vi "Gen Main.vi"(10 "Data Type DVRs":T1, 11 "Config Folder":path) -> ()   [LabVIEW 2018]
uses:
  <vilib>/ORNL/CSEISMIC DDS/CSEISMIC DDS Base/Data Types/Controls/DeviceID.ctl
  Controls/DDS State.ctl
  Controls/Data Type DVRs.ctl
  Controls/Generation Mode Loop Selector.ctl
  <vilib>/ORNL/CSEISMIC DDS/CSEISMIC DDS Base/Data Types/DER_setGenerationMode.ctl
  <vilib>/ORNL/CSEISMIC DDS/CSEISMIC DDS Base/Data Types/Controls/Generation Mode.ctl
  Controls/GenerationMode.ctl
  <vilib>/ORNL/CSEISMIC DDS/CSEISMIC DDS Base/Data Types/IED_Status.ctl
  <vilib>/ORNL/CSEISMIC DDS/CSEISMIC DDS Base/Data Types/Controls/Timestamp.ctl
  <vilib>/ORNL/CSEISMIC DDS/CSEISMIC DDS Base/Data Types/DER_Control.ctl
  <vilib>/ORNL/CSEISMIC DDS/CSEISMIC DDS Base/Data Types/DER_SetPointP.ctl
  <vilib>/ORNL/CSEISMIC DDS/CSEISMIC DDS Base/Data Types/DER_SetPointQ.ctl
  <vilib>/ORNL/CSEISMIC DDS/CSEISMIC DDS Base/Data Types/DER_SetPointF.ctl
  <vilib>/ORNL/CSEISMIC DDS/CSEISMIC DDS Base/Data Types/DER_VF.ctl
  <vilib>/ORNL/CSEISMIC DDS/CSEISMIC DDS Base/Data Types/DER_SetPointV.ctl
  <vilib>/ORNL/CSEISMIC DDS/CSEISMIC DDS Base/Data Types/DER_Measurement.ctl
  <vilib>/ORNL/CSEISMIC DDS/CSEISMIC DDS Base/Data Types/DER_Status.ctl
  <vilib>/ORNL/CSEISMIC DDS/CSEISMIC DDS Base/Data Types/Controls/DroopCurve.ctl
  401ef75d-4035-4dac-a689-94d2924f7ced.vi
  ab331fe9-b04e-4426-a1fd-c0893e9cbbab.vi
  3f4c0bec-be85-4757-afce-5fb011e1cb8b.vi
  89cbe241-b989-4977-afe6-711c5348a61b.vi
  9317fa08-e0dc-4cca-bb56-0a6db7703743.vi
  886c343d-5278-4dca-8794-94646f0fb70e.vi
  c2bfef2e-7af0-43a2-a662-0b996137247f.vi
  dc0c45d3-0bd6-4f4b-910c-54dfdd797161.vi
  e30d74d1-6a2d-4639-bc13-a8367489f367.vi
  906873a0-33da-4e1e-a43f-91631b103c02.vi
  1debb0a8-2f31-4473-8656-42ab50186c7a.vi
  21a46faf-e81a-4fcd-8f80-ead2e695587f.vi
  38cde540-623b-4de9-a38b-94f214654436.vi
  4f1983b4-d265-4997-ba90-a7128872a41b.vi
  66ace3ea-5fe4-466d-8ac4-009297ea2c08.vi
  Global Variables/Stop (Global).vi
  Global Variables/Measurements (Global).vi
  Global Variables/DDS States (Global).vi
  <vilib>/ORNL/CSEISMIC DDS/CSEISMIC DDS Base/CSEISMIC DDS.lvclass
panel:
  out "P_ref":sgl
  out "Q_ref":sgl
  out "P_meas":sgl
  out "Vf Control":bool
  out "Q_meas":sgl
  out "f_islanded":fxp<+,20,6>
  out "Vq_ref":sgl
  out "Is VF Device?":bool
  in  "Ramp Rate (W)":sgl=5000.0
  out "MicrogridID":u8
  out "Error in DDS Loop":bool
  out "DDS Loop error out":errorcluster
  out "DDS State":T2=enum."Shutdown"
  out "DDS loop time":u32=103
  out "DDS Indicators":T3
  out "Error in Generation Mode Loop":bool
  out "error out GenMode Loop":errorcluster
  out "DDS state m/c loop time":u32=100
  out "DeviceID":T4
  out "Enable INV A":bool
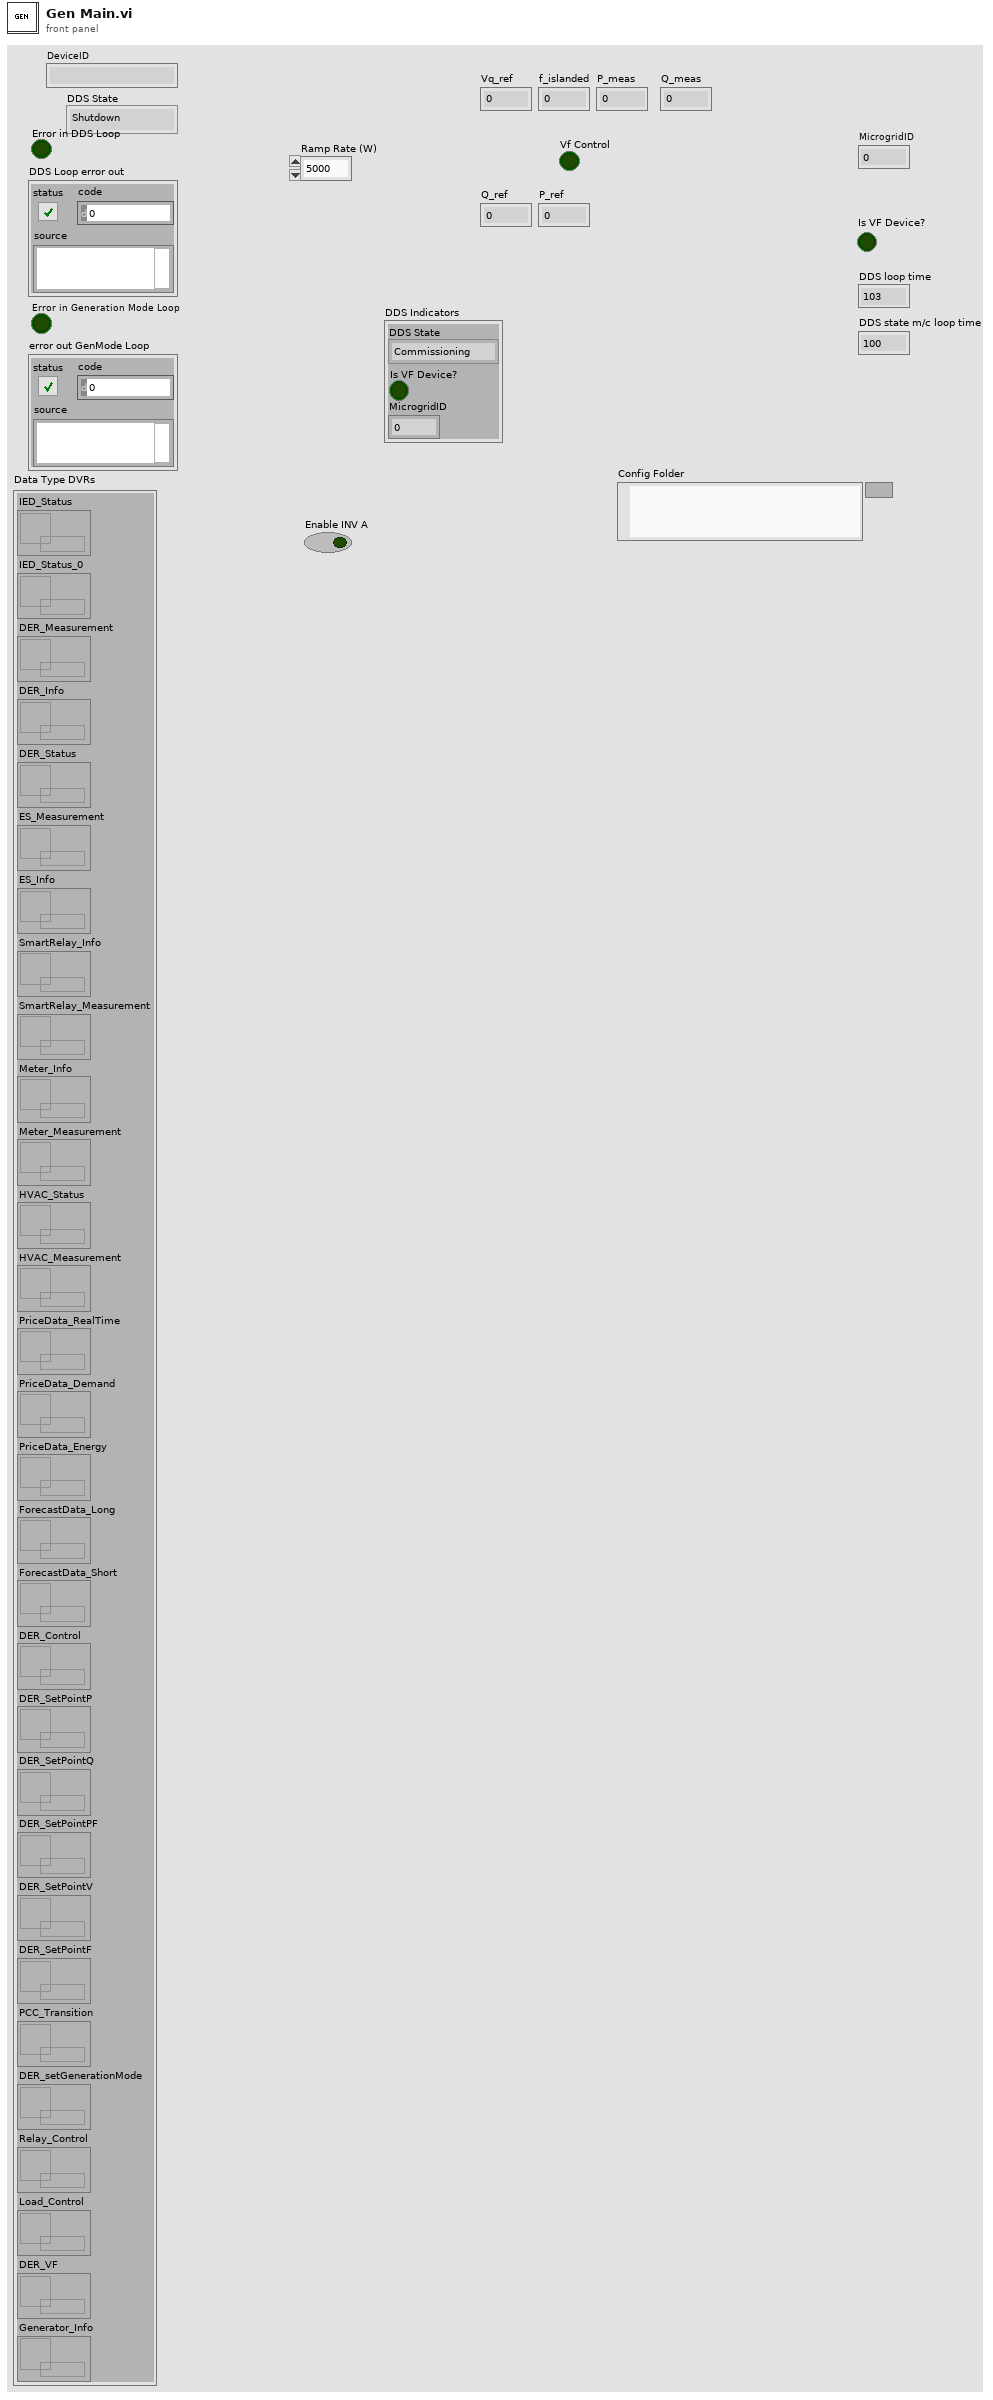
[diagram p1: front panel]
types:
  T1 = typedef "Data Type DVRs.ctl" = cluster{"IED_Status":refnum<data-value>, "IED_Status_0":refnum<data-value>, "DER_Measurement":refnum<data-value>, "DER_Info":refnum<data-value>, "DER_Status":refnum<data-value>, "ES_Measurement":refnum<data-value>, "ES_Info":refnum<data-value>, "SmartRelay_Info":refnum<data-value>, "SmartRelay_Measurement":refnum<data-value>, "Meter_Info":refnum<data-value>, "Meter_Measurement":refnum<data-value>, "HVAC_Status":refnum<data-value>, "HVAC_Measurement":refnum<data-value>, "PriceData_RealTime":refnum<data-value>, "PriceData_Demand":refnum<data-value>, "PriceData_Energy":refnum<data-value>, "ForecastData_Long":refnum<data-value>, "ForecastData_Short":refnum<data-value>, "DER_Control":refnum<data-value>, "DER_SetPointP":refnum<data-value>, "DER_SetPointQ":refnum<data-value>, "DER_SetPointPF":refnum<data-value>, "DER_SetPointV":refnum<data-value>, "DER_SetPointF":refnum<data-value>, "PCC_Transition":refnum<data-value>, "DER_setGenerationMode":refnum<data-value>, "Relay_Control":refnum<data-value>, "Load_Control":refnum<data-value>, "DER_VF":refnum<data-value>, "Generator_Info":refnum<data-value>}
  T2 = typedef "DDS State.ctl" = enum16{"Commissioning", "CheckID", "InitDDS", "ReadDDS", "WriteDDS", "CheckClose", "Close", "Shutdown"}
  T3 = cluster{"DDS State":T2, "Is VF Device?":bool, "MicrogridID":u8}
  T4 = typedef "CSEISMIC DDS.lvlib/CSEISMIC DDS.lvclass/DeviceID.ctl" = string
  T5 = typedef "Generation Mode Loop Selector.ctl" = enum16{"Commissioning", "Start", "Active", "VF Device", "Hold", "Close References", "Shutdown"}
  T6 = typedef "Scaling Coefficients Cluster.ctl" = cluster{"Measurements":T7, "Setpoints":T8}
  T7 = typedef "Scaling Coefficients Measurements.ctl" = cluster{"Current":dbl, "Voltage":dbl, "Real Power":dbl, "Reactive Power":dbl, "SOC":dbl}
  T8 = typedef "Scaling Coefficients Setpoints.ctl" = cluster{"Voltage":dbl, "Frequency":dbl, "Real Power":dbl, "Reactive Power":dbl}
  T9 = typedef "CSEISMIC DDS.lvlib/CSEISMIC DDS.lvclass/DER_Info.ctl" = cluster{"DeviceID":T4, "LineConfig":u8[], "NominalVoltage(V)":dbl, "PowerRating(kVA)":dbl, "VFControl":bool, "PControl":bool, "QControl":bool, "PFControl":bool, "PVControl":bool, "Droop":bool, "DroopConfigurable":bool, "Unbalanced":bool}
  T10 = typedef "CSEISMIC DDS.lvlib/CSEISMIC DDS.lvclass/Generator_Info.ctl" = cluster{"DeviceID":T4, "Voltage (V)":dbl, "MinimumPower (kVA)":dbl, "EnergyRating (kWh)":dbl, "RampRate (kW/s)":dbl, "MaxPowerFactorLeading":dbl, "MaxPowerFactorLagging":dbl, "EfficiencyCurve":T11, "StartCost":dbl, "FuelCost":dbl, "StartTime (s)":dbl}
  T11 = typedef "CSEISMIC DDS.lvlib/CSEISMIC DDS.lvclass/EfficiencyCurve.ctl" = cluster{"Power (kW)":dbl[], "Efficiency (%)":dbl[]}
  T12 = typedef "CSEISMIC DDS.lvlib/CSEISMIC DDS.lvclass/DER_setGenerationMode.ctl" = cluster{"DeviceID":T4, "Mode":T13}
  T13 = typedef "CSEISMIC DDS.lvlib/CSEISMIC DDS.lvclass/Generation Mode.ctl" = enum32{"Invalid", "PQ", "Droop", "PV", "PF", "VF"}
  T14 = typedef "GenerationMode.ctl" = enum32{"Invalid", "PQ", "Droop", "PV", "PF", "VF"}
  T15 = typedef "CSEISMIC DDS.lvlib/CSEISMIC DDS.lvclass/Timestamp.ctl" = cluster{"Seconds":u64, "Remainder":u64}
  T16 = typedef "CSEISMIC DDS.lvlib/CSEISMIC DDS.lvclass/IED_Status.ctl" = cluster{"DeviceID":T4, "Timestamp":T15, "MicrogridID":u8, "Active":bool, "Inactive":bool, "Error":i32, "Fault":bool, "ErrorString":string}
  T17 = typedef "CSEISMIC DDS.lvlib/CSEISMIC DDS.lvclass/DER_SetPointV.ctl" = cluster{"DeviceID":T4, "Voltage (V)":dbl}
  T18 = typedef "CSEISMIC DDS.lvlib/CSEISMIC DDS.lvclass/DER_VF.ctl" = cluster{"DeviceID":T4}
  T19 = typedef "CSEISMIC DDS.lvlib/CSEISMIC DDS.lvclass/DER_SetPointF.ctl" = cluster{"DeviceID":T4, "Frequency (Hz)":dbl}
  T20 = typedef "CSEISMIC DDS.lvlib/CSEISMIC DDS.lvclass/DER_SetPointQ.ctl" = cluster{"DeviceID":T4, "ReactivePower (kVAR)":dbl[]}
  T21 = typedef "CSEISMIC DDS.lvlib/CSEISMIC DDS.lvclass/DER_SetPointP.ctl" = cluster{"DeviceID":T4, "RealPower (kW)":dbl[]}
  T22 = typedef "CSEISMIC DDS.lvlib/CSEISMIC DDS.lvclass/DER_Control.ctl" = cluster{"DeviceID":T4, "Activate":bool, "Deactivate":bool}
  T23 = typedef "CSEISMIC DDS.lvlib/CSEISMIC DDS.lvclass/DER_Status.ctl" = cluster{"DeviceID":T4, "VFControl":bool, "PControl":bool, "QControl":bool, "PFControl":bool, "PVControl":bool, "Droop":bool, "Unbalanced":bool, "MicrogridVF":bool, "RealDroop(kW)":T24, "ReactiveDroop(kVar)":T24}
  T24 = typedef "CSEISMIC DDS.lvlib/CSEISMIC DDS.lvclass/DroopCurve.ctl" = cluster{"XMin":dbl, "XMax":dbl, "YMin":dbl, "YMax":dbl}
  T25 = typedef "CSEISMIC DDS.lvlib/CSEISMIC DDS.lvclass/DER_Measurement.ctl" = cluster{"DeviceID":T4, "Voltage":dbl[], "Current":dbl[], "RealPower":dbl[], "ReactivePower":dbl[], "LineConfig":u8[], "Frequency":dbl}
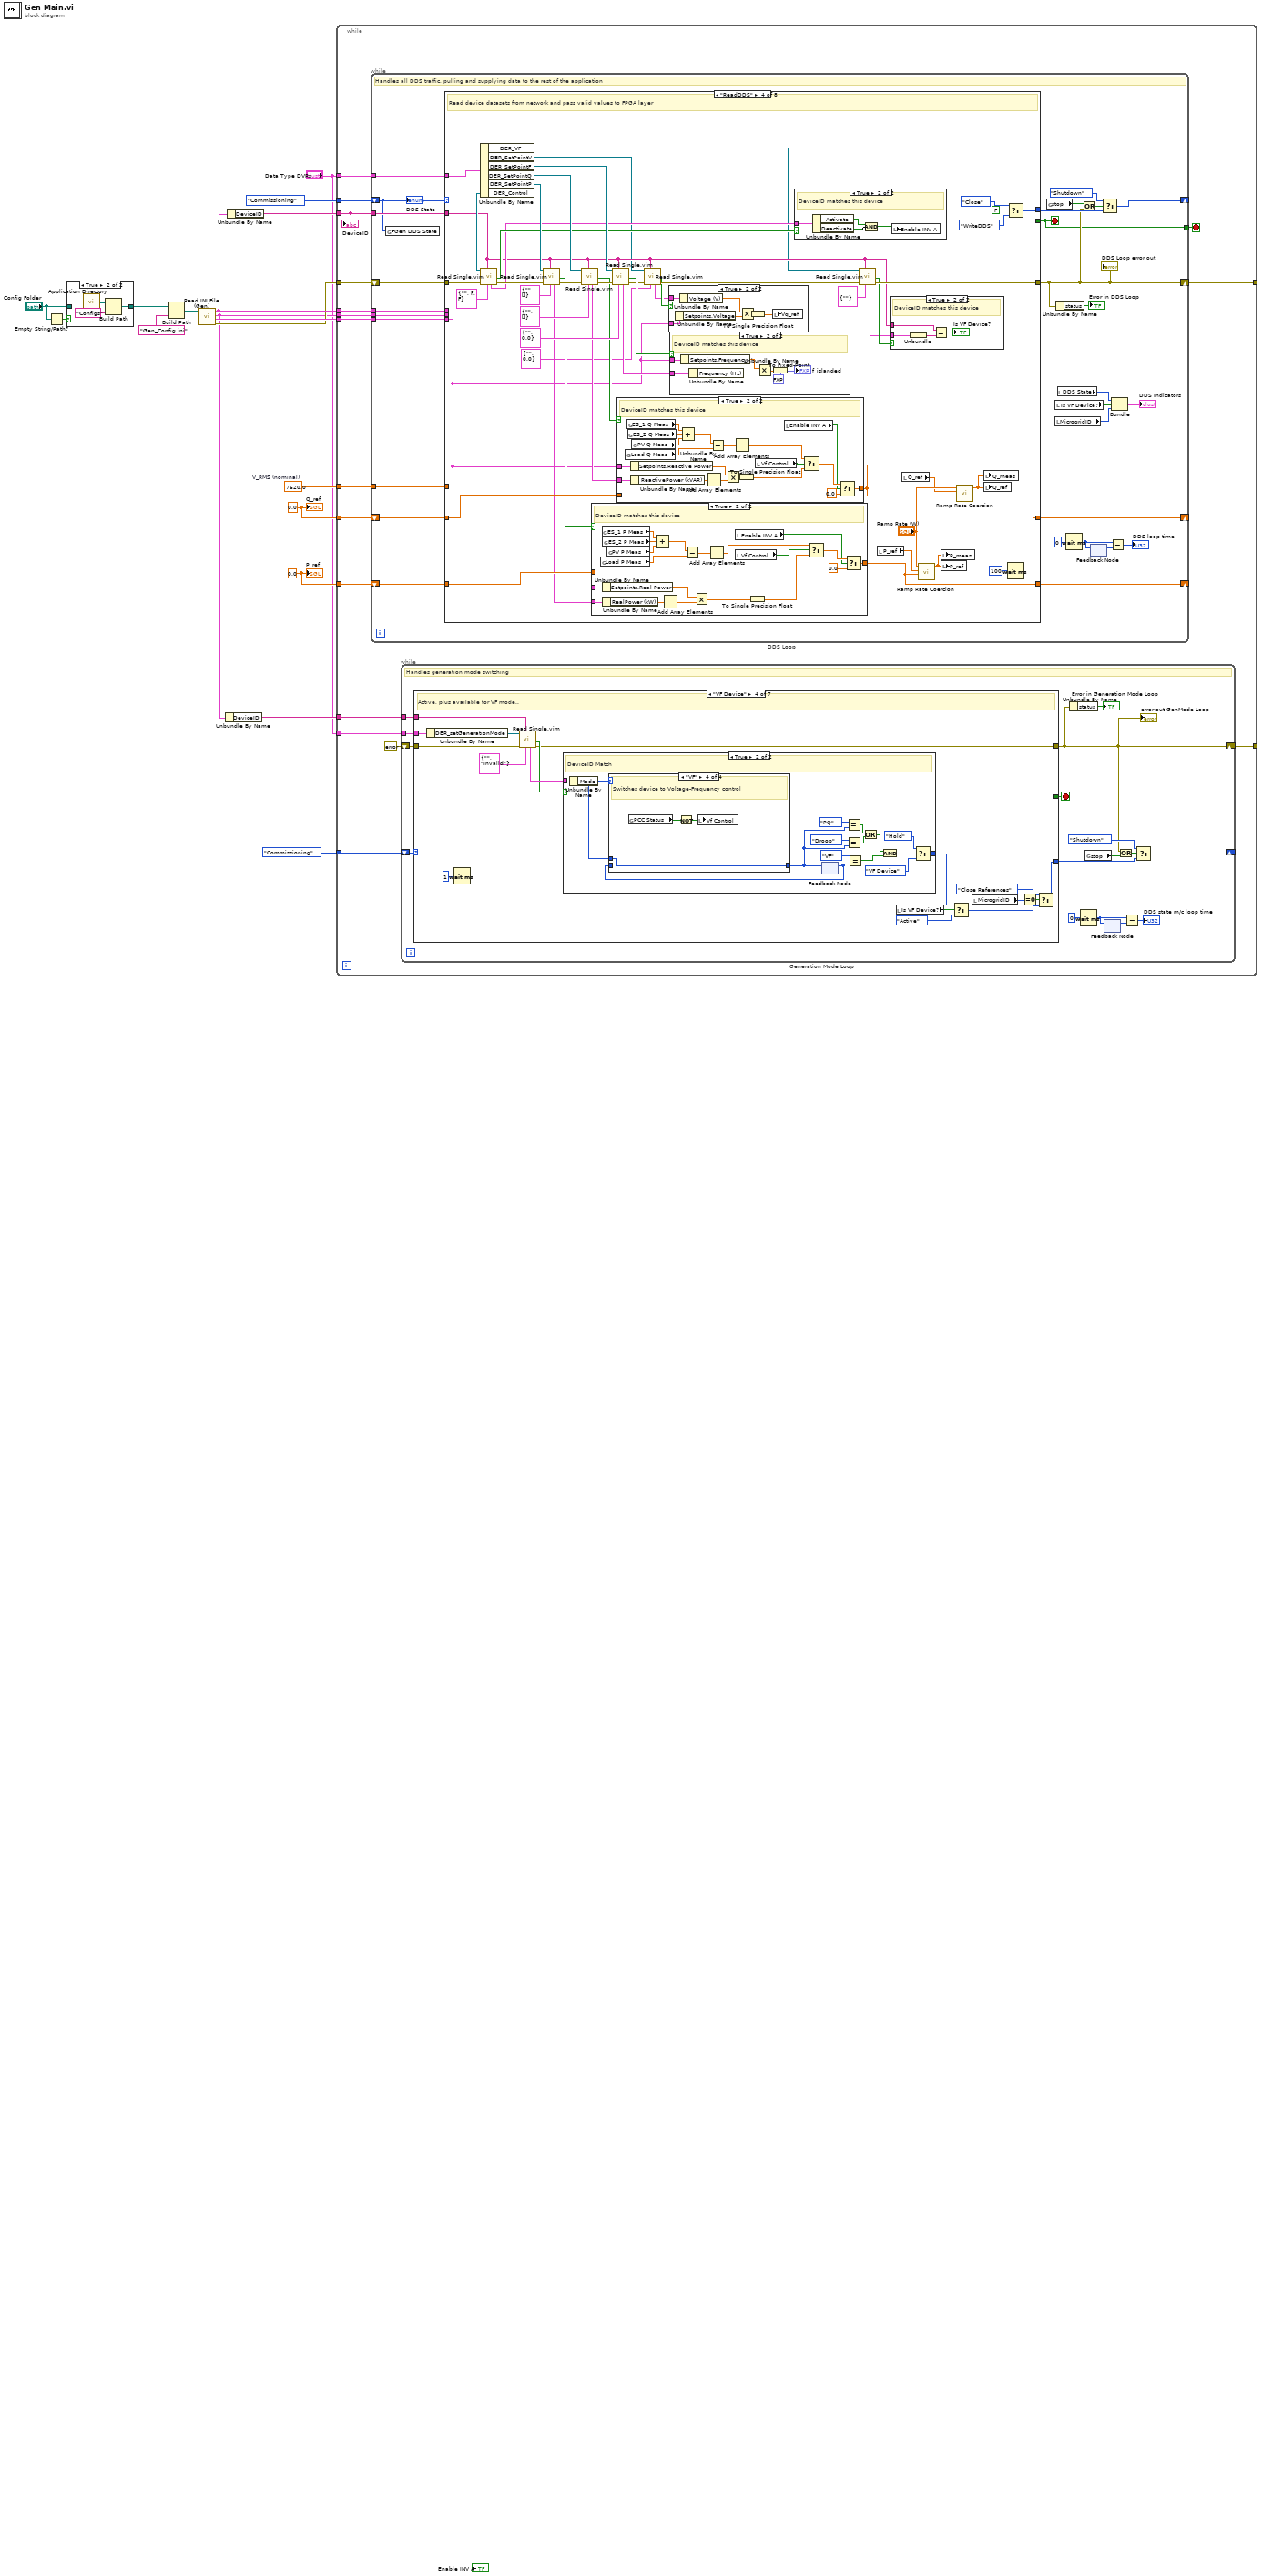
[diagram p0: block diagram]
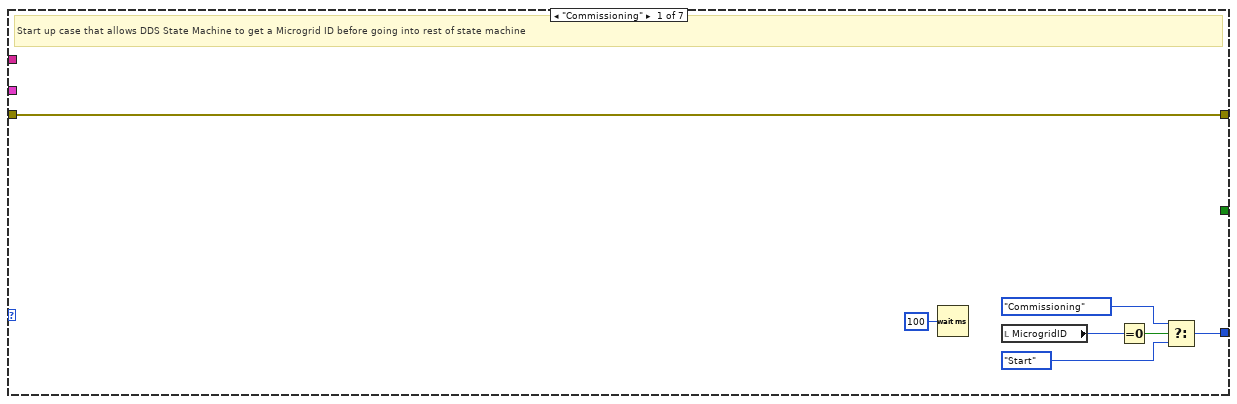
[diagram p2: hidden frame]
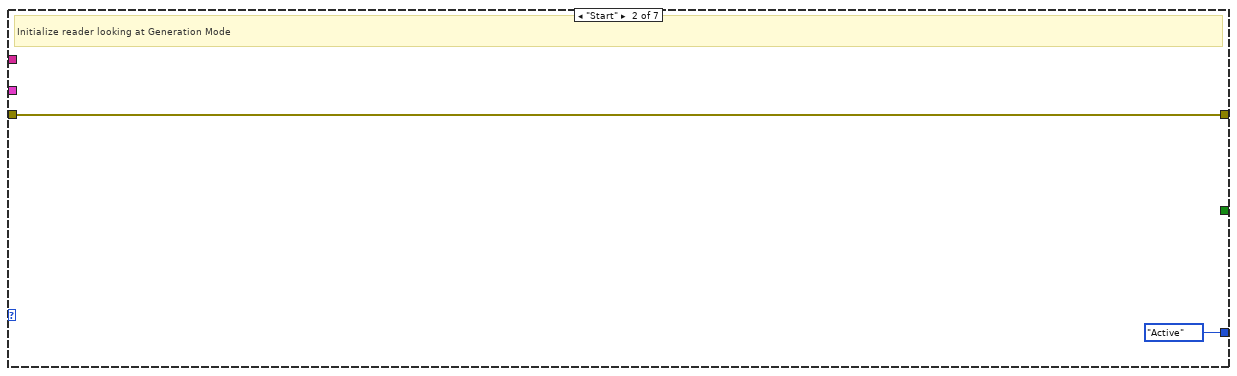
[diagram p3: hidden frame]
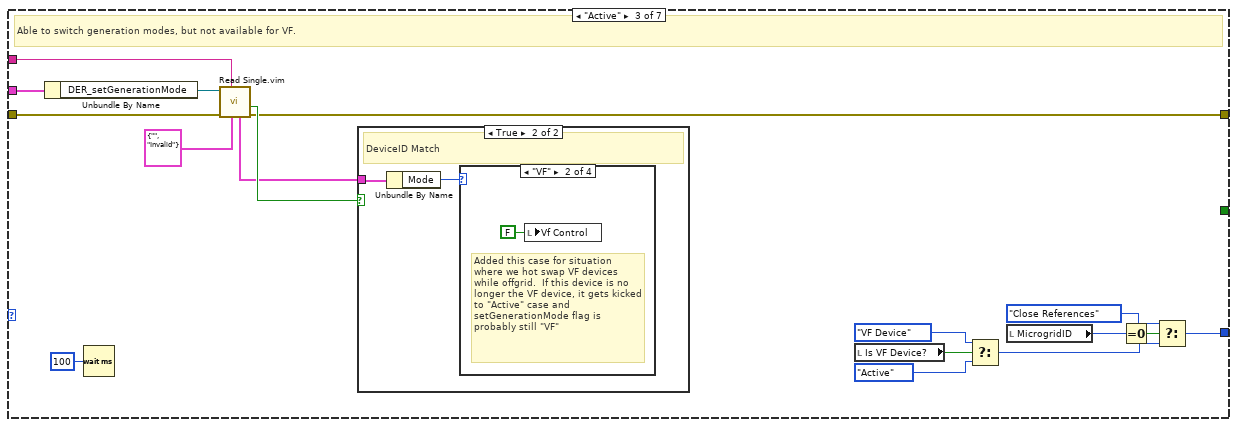
[diagram p4: hidden frame]
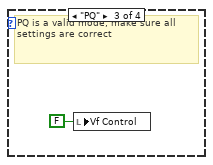
[diagram p7: hidden frame]
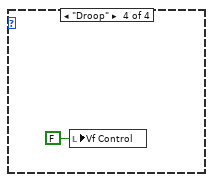
[diagram p8: hidden frame]
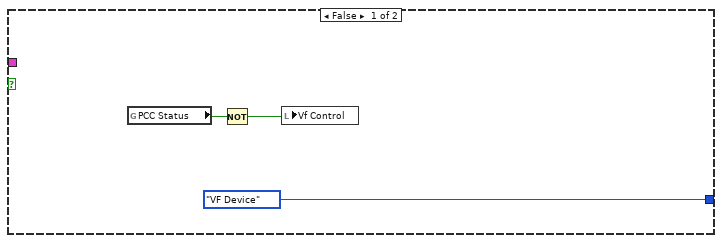
[diagram p9: hidden frame]
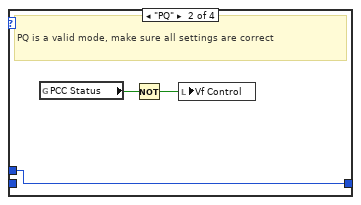
[diagram p11: hidden frame]
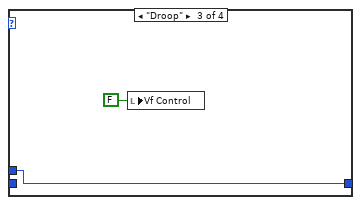
[diagram p12: hidden frame]
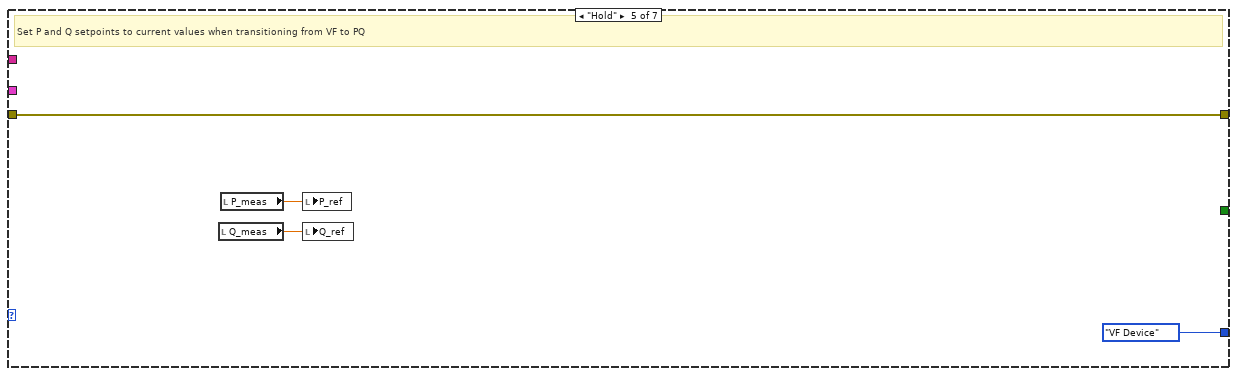
[diagram p13: hidden frame]
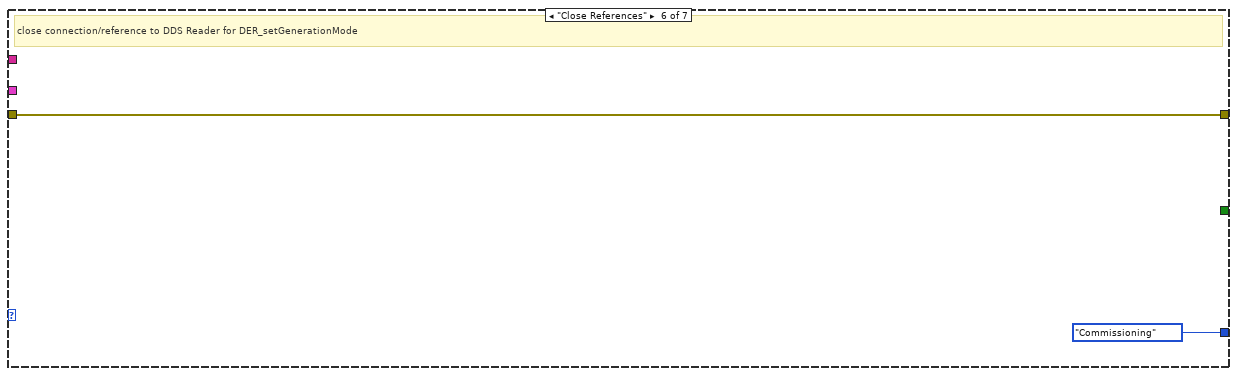
[diagram p14: hidden frame]
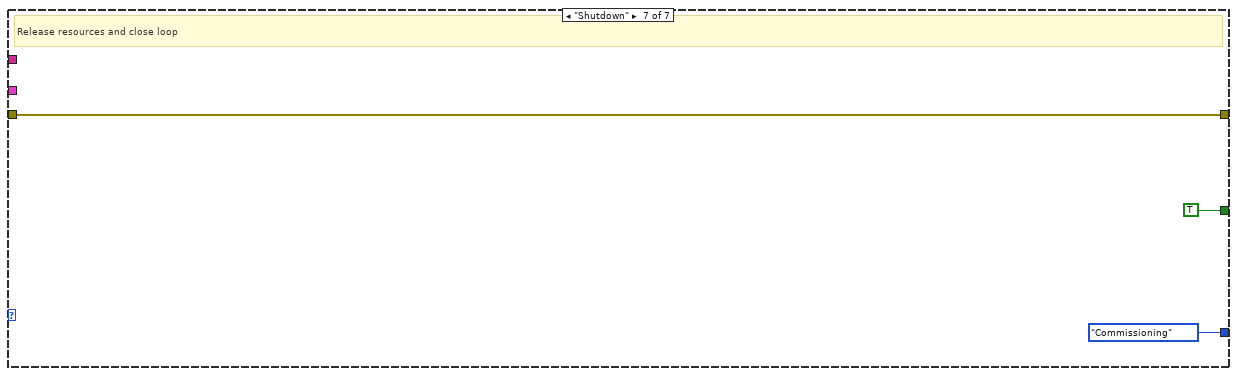
[diagram p15: hidden frame]
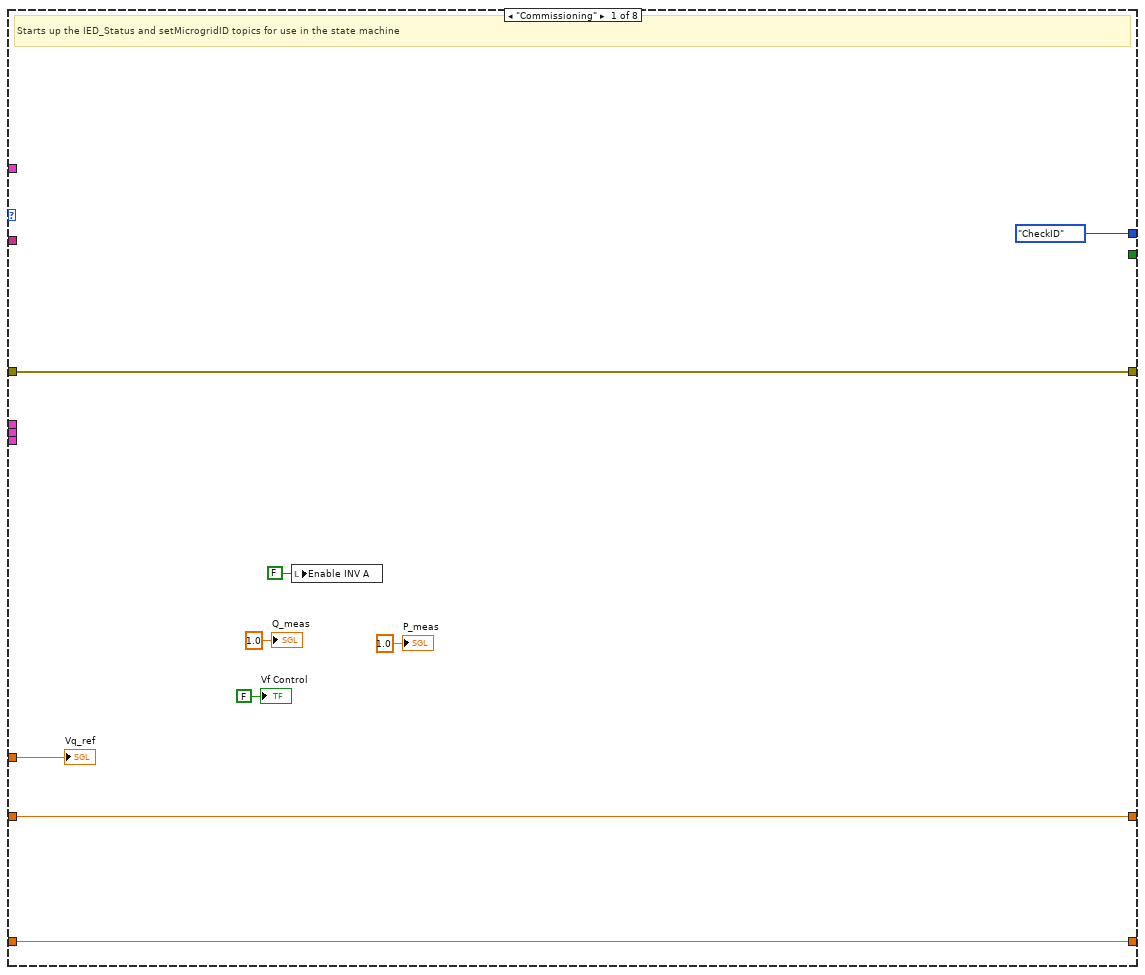
[diagram p16: hidden frame]
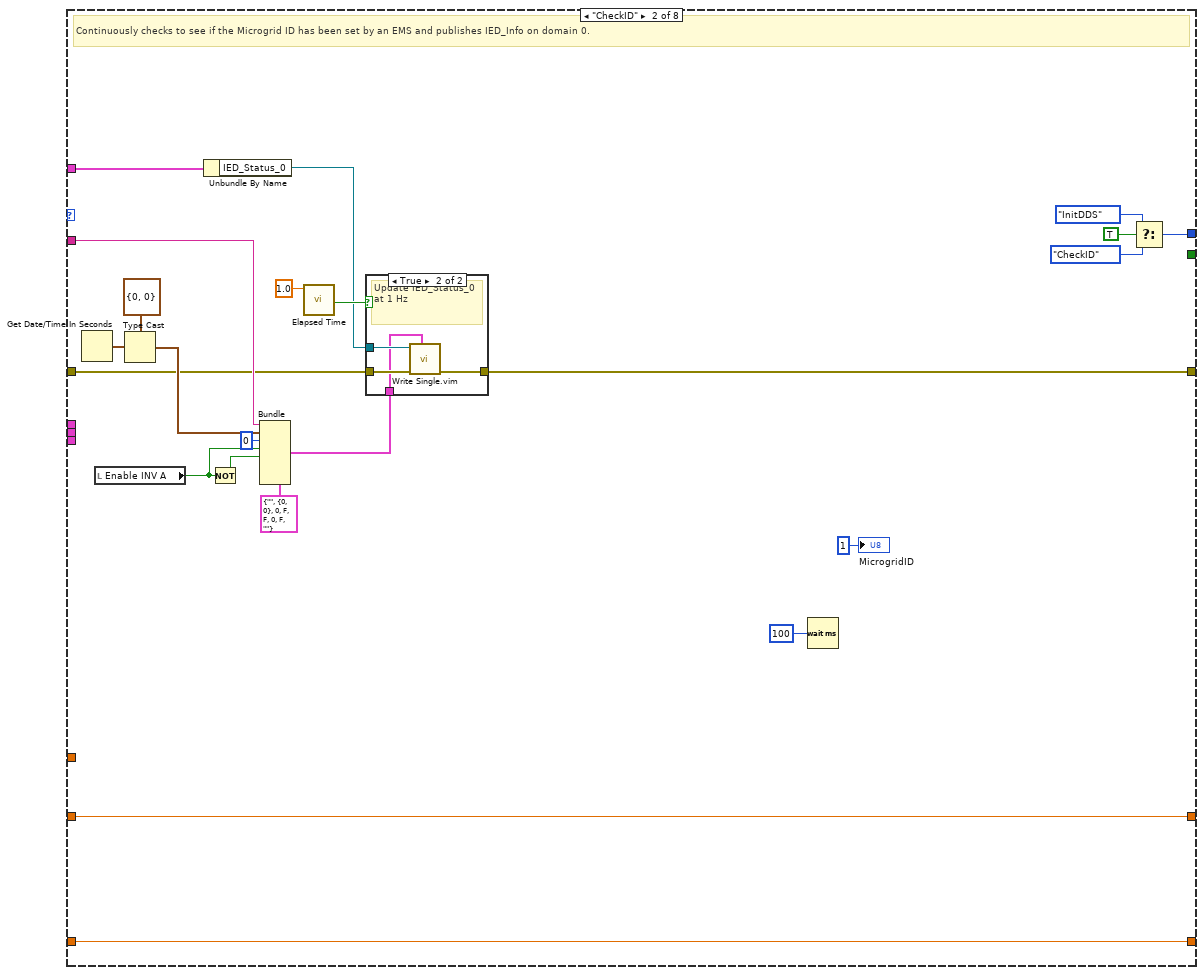
[diagram p17: hidden frame]
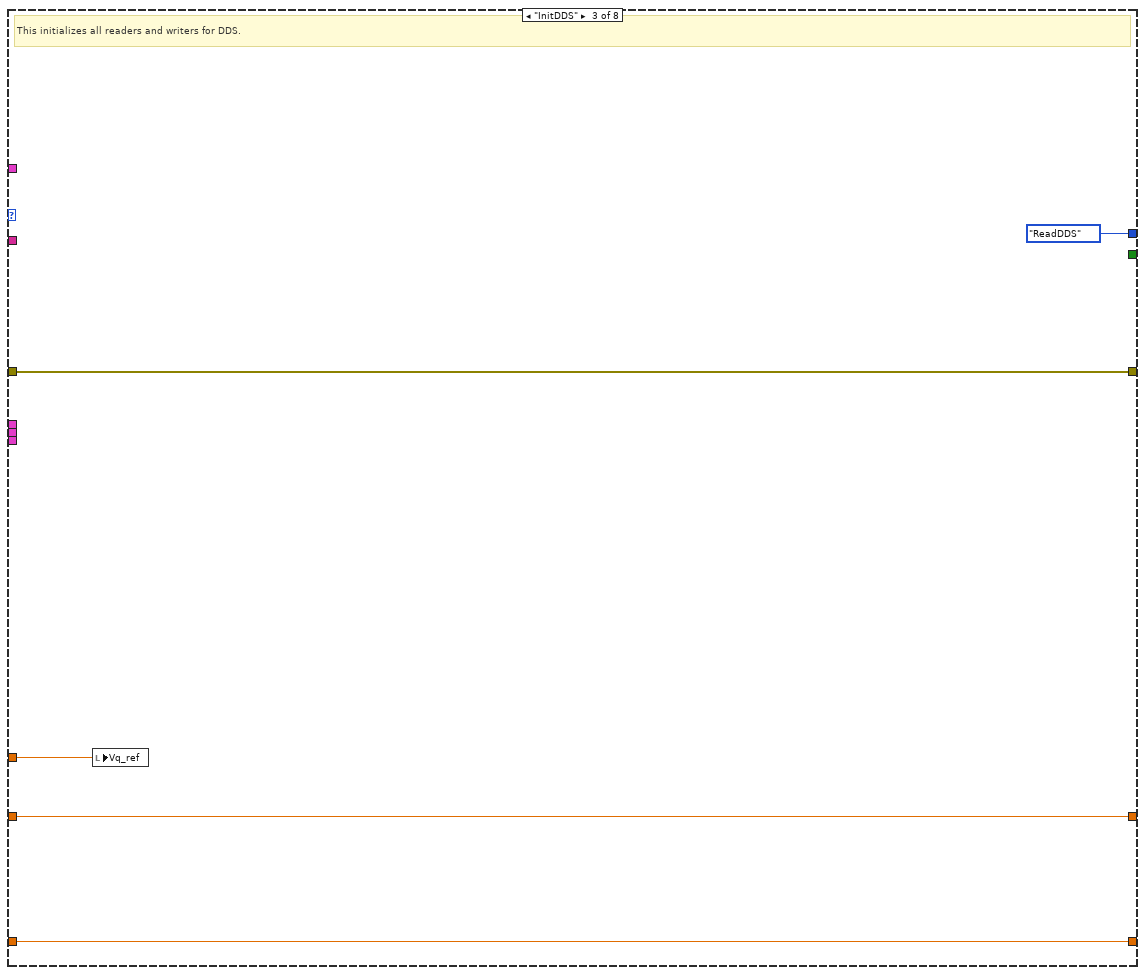
[diagram p19: hidden frame]
diagram:
  w5 = 7620.0  # V_RMS (nominal)
  w6 = sgl 0.0 ("Q_ref")
  w7 = sgl 0.0 ("P_ref")
  n1 = Empty String/Path?(string/path="Config Folder") -> (empty?=w4:bool)
  n2 = case shown="True" w4 {
    tunnel: [w18 w19] -> w2
    tunnel: "Config Folder" -> [w18 _]
    frame False {
    }
    frame True {
      n3 = call <vilib>:"Application Directory.vi"() -> ("Application Directory"=w21:path)
      n4 = Build Path(base path=w21, name or relative path="Configs") -> (appended path=w19:path)
    }
  }
  n5 = Build Path(base path=w2, name or relative path="Gen_Config.ini") -> (appended path=w16:path)
  n6 = call "Read INI File (Gen).vi"("Path"=w16) -> ("error out"=w12:errorcluster, "Scaling Coefficients"=w13:T6, "DER_Info"=w10:T9, "Generator_Info"=w14:T10)  [unwired: 7 in]
  n7 = Unbundle By Name(w10) -> ("DeviceID"=w11:T4)
  n8 = Unbundle By Name(w14) -> ("DeviceID"=w15:T4)
  n9 = while {
    tunnel: DDS_State."Commissioning" ("DDS State 2") -> [w38]
    tunnel: w10 -> [w37]
    tunnel: w12 -> [w36]
    tunnel: w13 -> [w35]
    tunnel: w15 -> [w34]
    tunnel: w14 -> [w33]
    tunnel: w11 -> [w31]
    tunnel: Generation_Mode_Loop_Selector."Commissioning" -> [w30]
    tunnel: [w29] -> _
    tunnel: [w28] -> _
    tunnel: w7 -> [w27]
    tunnel: w6 -> [w26]
    tunnel: w5 -> [w25]
    tunnel: "Data Type DVRs" -> [w24]
    tunnel: "Data Type DVRs" -> [w23]
    stop <- w32 stop-if-true
    n10 = while "DDS Loop" {
      shift-right: [w161] -> _
      shift-left: w38 -> [w139]
      tunnel: w34 -> [w165]
      shift-right: [w156] -> w28
      shift-left: w36 -> [w164]
      tunnel: w33 -> [w163]
      tunnel: w37 -> [w162]
      tunnel: w35 -> [w157]
      tunnel: [w154] -> w32
      shift-right: [w149] -> _
      shift-left: w27 -> [w148]
      shift-right: [w147] -> _
      shift-left: w26 -> [w146]
      tunnel: w25 -> [w141]
      tunnel: w24 -> [w166]
      stop <- w154 stop-if-true
      # "Handles all DDS traffic, pulling and supplying data to the rest of the application"
      n11 = global write "DDS States (Global).vi" "Gen DDS State"(w139) -> ()
      n12 = case shown="\"ReadDDS\"" w139 {
        tunnel: [DDS_State."CheckID" w195 DDS_State."ReadDDS" w254 DDS_State."CheckClose" w424 DDS_State."Commissioning" ("f") DDS_State."Commissioning" ("f")] -> w160
        tunnel: w166 -> [_ w178 _ w231 w333 _ _ _]
        tunnel: [w174 w181 w207 w229 w326 w423 w430 w437] -> w156
        tunnel: w165 -> [_ w187 _ w215 w360 _ _ _]
        tunnel: w164 -> [w174 w182 w207 w232 w334 w423 w430 w437]
        tunnel: w163 -> [_ _ _ _ w329 _ _ _]
        tunnel: w162 -> [_ _ _ _ w328 _ _ _]
        tunnel: [_ _ _ _ _ _ _ TRUE] -> w154
        tunnel: w157 -> [_ _ _ w209 w374 _ _ _]
        tunnel: [w173 w186 w206 w252 w356 w422 w428 w434] -> w149
        tunnel: w148 -> [w173 w186 w206 w251 w356 w422 w428 w434]
        tunnel: [w172 w185 w205 w249 w355 w421 w427 w433] -> w147
        tunnel: w146 -> [w172 w185 w205 w248 w355 w421 w427 w433]
        tunnel: w141 -> [w167 _ w204 _ w346 _ _ _]
        frame "Commissioning" {
          # "Starts up the IED_Status and setMicrogridID topics for use in the state machine"
          n13 = local write "Enable INV A"(FALSE ("Enable INV A")) -> ()
          "Q_meas" <- sgl 1.0 ("Q_meas")
          "Vf Control" <- FALSE ("Vf Control")
          "P_meas" <- sgl 1.0 ("P_meas")
          "Vq_ref" <- w167
        }
        frame "CheckID" {
          # "Continuously checks to see if the Microgrid ID has been set by an EMS and publishes IED_Info on domain 0."
          n14 = Get Date/Time In Seconds() -> (seconds since 1Jan1904=w192:timestamp)
          n15 = local read "Enable INV A"() -> (w184:bool)
          n16 = Type Cast(type=T15 {"Seconds"=0, "Remainder"=0} ("Timestamp"), x=w192) -> (*(type *) &x=w190:T15)
          n17 = Unbundle By Name(w178) -> ("IED_Status_0"=w179:refnum<data-value>)
          n18 = Not(x=w184) -> (.not. x?=w188:bool)
          n19 = Bundle(cluster=T16 {"DeviceID"="", "Timestamp"={"Seconds"=0, "Remainder"=0}, "MicrogridID"=0, "Active"=FALSE, "Inactive"=FALSE, "Error"=0, "Fault"=FALSE, "ErrorString"=""} ("output cluster"), "DeviceID"=w187, "Timestamp"=w190, "MicrogridID"=u8 0, "Active"=w184, "Inactive"=w188) -> (w180:T16)  [unwired: 3 in]
          n20 = call "Elapsed Time"("Time Target (s)"=1.0) -> ("Time has Elapsed"=w183:bool)  [unwired: 11 in, 7 out]
          n21 = case shown="True" w183 {
            tunnel: w180 -> [_ w200]
            tunnel: [w199 w201] -> w181
            tunnel: w182 -> [w199 w202]
            tunnel: w179 -> [_ w203]
            frame False {
            }
            frame True {
              # "Update IED_Status_0 at 1 Hz"
              n22 = call "Write Single.vim"("Data Element"=w200, "error in"=w202, "Data DVR"=w203) -> ("dup error out"=w201:errorcluster)  [unwired: 8 in]
            }
          }
          n23 = Wait (ms)(milliseconds to wait=u32 100) -> ()  [unwired: 1 out]
          n24 = Select(t=DDS_State."InitDDS", s=TRUE, f=DDS_State."CheckID") -> (s? t:f=w195:T2)
          "MicrogridID" <- u8 1 ("MicrogridID")
        }
        frame "InitDDS" {
          # "This initializes all readers and writers for DDS."
          n25 = local write "Vq_ref"(w204) -> ()
        }
        frame "ReadDDS" {
          # "Read device datasets from network and pass valid values to FPGA layer"
          n26 = Unbundle By Name(w231) -> ("DER_VF"=w214:refnum<data-value>, "DER_SetPointV"=w213:refnum<data-value>, "DER_SetPointF"=w241:refnum<data-value>, "DER_SetPointQ"=w239:refnum<data-value>, "DER_SetPointP"=w237:refnum<data-value>, "DER_Control"=w233:refnum<data-value>)
          n27 = call "Read Single.vim"("Data Type"=T22 {"DeviceID"="", "Activate"=FALSE, "Deactivate"=FALSE} ("DER_Control"), "DeviceID"=w215, "error in"=w232, "Data DVR"=w233) -> ("dup error out"=w235:errorcluster, "Valid"=w225:bool, "Data Element"=w224:T22)  [unwired: 5 in]
          n28 = call "Read Single.vim"("Data Type"=T21 {"DeviceID"="", "RealPower (kW)"=[]} ("DER_SetPointP"), "DeviceID"=w215, "error in"=w235, "Data DVR"=w237) -> ("dup error out"=w238:errorcluster, "Valid"=w223:bool, "Data Element"=w222:T21)  [unwired: 5 in]
          n29 = call "Read Single.vim"("Data Type"=T20 {"DeviceID"="", "ReactivePower (kVAR)"=[]} ("DER_SetPointQ"), "DeviceID"=w215, "error in"=w238, "Data DVR"=w239) -> ("dup error out"=w243:errorcluster, "Valid"=w221:bool, "Data Element"=w220:T20)  [unwired: 5 in]
          n30 = case shown="True" w223 {
            tunnel: w222 -> [_ w314]
            tunnel: w209 -> [_ w313]
            tunnel: [w295 w308] -> w252
            tunnel: w251 -> [w295 _]
            frame False {
              # "Non-matching DeviceID"
            }
            frame True {
              # "DeviceID matches this device"
              n31 = global read "Measurements (Global).vi" "Load P Meas"() -> (w301:dbl[])
              n32 = global read "Measurements (Global).vi" "ES_1 P Meas"() -> (w297:dbl[])
              n33 = Unbundle By Name(w313) -> ("Setpoints.Real Power"=w311:dbl)
              n34 = Unbundle By Name(w314) -> ("RealPower (kW)"=w312:dbl[])
              n35 = global read "Measurements (Global).vi" "ES_2 P Meas"() -> (w298:dbl[])
              n36 = global read "Measurements (Global).vi" "PV P Meas"() -> (w299:dbl[])
              n37 = Compound Arithmetic op=ADD(w297, w298, w299) -> (w300:dbl[])
              n38 = Add Array Elements(numeric array=w312) -> (sum=w310:dbl)
              n39 = Subtract(x=w300, y=w301) -> (x-y=w302:dbl[])
              n40 = Multiply(x=w311, y=w310) -> (x*y=w309:dbl)
              n41 = Add Array Elements(numeric array=w302) -> (sum=w296:dbl)
              n42 = local read "Enable INV A"() -> (w303:bool)
              n43 = local read "Vf Control"() -> (w304:bool)
              n44 = To Single Precision Float(number=w309) -> (single precision float=w306:sgl)
              n45 = Select(t=w296, s=w304, f=w306) -> (s? t:f=w305:dbl)
              n46 = Select(t=w305, s=w303, f=sgl 0.0) -> (s? t:f=w308:dbl)
            }
          }
          n47 = call "Read Single.vim"("Data Type"=T19 {"DeviceID"="", "Frequency (Hz)"=0.0} ("DER_SetPointVF"), "DeviceID"=w215, "error in"=w243, "Data DVR"=w241) -> ("dup error out"=w217:errorcluster, "Valid"=w219:bool, "Data Element"=w218:T19)  [unwired: 5 in]
          n48 = case shown="True" w221 {
            tunnel: w220 -> [_ w294]
            tunnel: w209 -> [_ w293]
            tunnel: [w275 w285] -> w249
            tunnel: w248 -> [w275 _]
            frame False {
              # "Non-matching DeviceID"
            }
            frame True {
              # "DeviceID matches this device"
              n49 = global read "Measurements (Global).vi" "Load Q Meas"() -> (w278:dbl[])
              n50 = global read "Measurements (Global).vi" "ES_1 Q Meas"() -> (w282:dbl[])
              n51 = global read "Measurements (Global).vi" "ES_2 Q Meas"() -> (w281:dbl[])
              n52 = Unbundle By Name(w293) -> ("Setpoints.Reactive Power"=w290:dbl)
              n53 = Unbundle By Name(w294) -> ("ReactivePower (kVAR)"=w292:dbl[])
              n54 = global read "Measurements (Global).vi" "PV Q Meas"() -> (w280:dbl[])
              n55 = Compound Arithmetic op=ADD(w282, w281, w280) -> (w279:dbl[])
              n56 = Add Array Elements(numeric array=w292) -> (sum=w291:dbl)
              n57 = Subtract(x=w279, y=w278) -> (x-y=w277:dbl[])
              n58 = Multiply(x=w290, y=w291) -> (x*y=w289:dbl)
              n59 = Add Array Elements(numeric array=w277) -> (sum=w276:dbl)
              n60 = To Single Precision Float(number=w289) -> (single precision float=w288:sgl)
              n61 = local read "Vf Control"() -> (w283:bool)
              n62 = local read "Enable INV A"() -> (w284:bool)
              n63 = Select(t=w276, s=w283, f=w288) -> (s? t:f=w287:dbl)
              n64 = Select(t=w287, s=w284, f=sgl 0.0) -> (s? t:f=w285:dbl)
            }
          }
          n65 = call "Read Single.vim"("Data Type"=T17 {"DeviceID"="", "Voltage (V)"=0.0} ("DER_SetPointVF"), "DeviceID"=w215, "error in"=w217, "Data DVR"=w213) -> ("dup error out"=w216:errorcluster, "Valid"=w212:bool, "Data Element"=w211:T17)  [unwired: 5 in]
          n66 = case shown="True" w212 {
            tunnel: w211 -> [_ w261]
            tunnel: w209 -> [_ w260]
            frame False {
            }
            frame True {
              n67 = Unbundle By Name(w260) -> ("Setpoints.Voltage"=w259:dbl)
              n68 = Unbundle By Name(w261) -> ("Voltage (V)"=w258:dbl)
              n69 = Multiply(x=w258, y=w259) -> (x*y=w262:dbl)
              n70 = To Single Precision Float(number=w262) -> (single precision float=w257:sgl)
              n71 = local write "Vq_ref"(w257) -> ()
            }
          }
          n72 = case shown="True" w219 {
            tunnel: w218 -> [_ w274]
            tunnel: w209 -> [_ w273]
            frame False {
              # "Non-matching DeviceID"
            }
            frame True {
              # "DeviceID matches this device"
              n73 = Unbundle By Name(w273) -> ("Setpoints.Frequency"=w272:dbl)
              n74 = Unbundle By Name(w274) -> ("Frequency (Hz)"=w271:dbl)
              n75 = Multiply(x=w272, y=w271) -> (x*y=w269:dbl)
              n76 = To Fixed-Point(fixed-point type=fxp<+,20,6> 0.0 ("f_islanded"), number=w269) -> (fixed-point=→"f_islanded":fxp<+,20,6>)
            }
          }
          n77 = case shown="True" w225 {
            tunnel: w224 -> [_ w318]
            frame False {
              # "Non-matching DeviceID"
            }
            frame True {
              # "DeviceID matches this device"
              n78 = Unbundle By Name(w318) -> ("Activate"=w316:bool, "Deactivate"=w317:bool)
              n79 = Compound Arithmetic op=AND(w316, invert w317) -> (w315:bool)
              n80 = local write "Enable INV A"(w315) -> ()
            }
          }
          n81 = call "Read Single.vim"("Data Type"=T18 {"DeviceID"=""} ("DER_VF"), "DeviceID"=w215, "error in"=w216, "Data DVR"=w214) -> ("dup error out"=w229:errorcluster, "Valid"=w228:bool, "Data Element"=w226:T18)  [unwired: 5 in]
          n82 = local read "P_ref"() -> (w246:sgl)
          n83 = case shown="True" w228 {
            tunnel: w226 -> [_ w267]
            tunnel: w215 -> [_ w265]
            frame False {
              # "Non-matching DeviceID"
              n84 = local write "Is VF Device?"(FALSE ("Is VF Device?")) -> ()
            }
            frame True {
              # "DeviceID matches this device"
              n85 = Unbundle(w267) -> ("DeviceID"=w266:T4)
              n86 = Equal?(x=w265, y=w266) -> (x = y?=→"Is VF Device?":bool)
            }
          }
          n87 = local read "Q_ref"() -> (w247:sgl)
          n88 = call "Ramp Rate Coercion.vi"("Requested Value"=w252, "Original Value"=w246, "Ramp Rate (W)"="Ramp Rate (W)") -> ("Coerced Value"=w245:sgl)  [unwired: 8 in]
          n89 = local write "P_meas"(w245) -> ()
          n90 = local write "P_ref"(w245) -> ()
          n91 = call "Ramp Rate Coercion.vi"("Requested Value"=w249, "Original Value"=w247, "Ramp Rate (W)"="Ramp Rate (W)") -> ("Coerced Value"=w244:sgl)  [unwired: 8 in]
          n92 = local write "Q_meas"(w244) -> ()
          n93 = local write "Q_ref"(w244) -> ()
          n94 = Wait (ms)(milliseconds to wait=u32 100) -> ()  [unwired: 1 out]
          n95 = Select(t=DDS_State."Close", s=FALSE, f=DDS_State."WriteDDS") -> (s? t:f=w254:T2)
        }
        frame "WriteDDS" {
          w359 = sgl 3.0 ("y")
          w349 = FALSE ("PFControl")
          # "#TODO add noise"
          # "Publish required datasets at required update rates to network"
          n96 = local read "Is VF Device?"() -> (w347:bool)
          n97 = Unbundle By Name(w333) -> ("DER_Status"=w320:refnum<data-value>, "DER_Measurement"=w322:refnum<data-value>, "IED_Status"=w324:refnum<data-value>, "IED_Status_0"=w330:refnum<data-value>, "Generator_Info"=w331:refnum<data-value>, "DER_Info"=w332:refnum<data-value>)
          n98 = Unbundle By Name(w328) -> ("LineConfig"=w377:u8[])
          n99 = Get Date/Time In Seconds() -> (seconds since 1Jan1904=w368:timestamp)
          n100 = local read "MicrogridID"() -> (w364:u8)
          n101 = Type Cast(type=T15 {"Seconds"=0, "Remainder"=0} ("Timestamp"), x=w368) -> (*(type *) &x=w365:T15)
          n102 = for {
            N: 3 -> [_]
            tunnel: [w409] -> w373 mode=indexing
            tunnel: [w408] -> w372 mode=indexing
            tunnel: w347 -> [w405]
            tunnel: w346 -> [w404]
            tunnel: [w403] -> w345
            # "#TODO add noise"
            n103 = case shown="True" w405 {
              tunnel: [w413 w418] -> w407
              tunnel: [w414 w419] -> w406
              tunnel: w404 -> [w413 _]
              tunnel: [fxp<+,20,6> 60.0 ("f_islanded") w417] -> w402
              frame False {
                n104 = local read "P_meas"() -> (w411:sgl)
                n105 = expression code="x*1000"(w411) -> (w410:sgl)
                n106 = Divide(x=w410, y=w413) -> (x/y=w414:dbl)
              }
              frame True {
                n107 = local read "P_meas"() -> (w416:sgl)
                n108 = local read "Vq_ref"() -> (w418:sgl)
                n109 = local read "f_islanded"() -> (w417:fxp<+,20,6>)
                n110 = expression code="x*1000"(w416) -> (w415:sgl)
                n111 = Divide(x=w415, y=w418) -> (x/y=w419:sgl)
              }
            }
            n112 = To Double Precision Float(number=w402) -> (double precision float=w403:dbl)
            n113 = To Double Precision Float(number=w407) -> (double precision float=w409:dbl)
            n114 = To Double Precision Float(number=w406) -> (double precision float=w408:dbl)
          }
          n115 = Unbundle By Name(w374) -> ("Measurements.Reactive Power"=w341:dbl, "Measurements.Real Power"=w343:dbl, "Measurements.Current"=w370:dbl, "Measurements.Voltage"=w371:dbl)
          n116 = local read "Enable INV A"() -> (w354:bool)
          n117 = call "Elapsed Time4"("Time Target (s)"=1.0) -> ("Time has Elapsed"=w375:bool)  [unwired: 11 in, 7 out]
          n118 = local read "Q_meas"() -> (w352:sgl)
          n119 = local read "P_meas"() -> (w353:sgl)
          n120 = Not(x=w354) -> (.not. x?=w363:bool)
          n121 = Bundle(cluster=T16 {"DeviceID"="", "Timestamp"={"Seconds"=0, "Remainder"=0}, "MicrogridID"=0, "Active"=FALSE, "Inactive"=FALSE, "Error"=0, "Fault"=FALSE, "ErrorString"=""} ("IED_Status"), "DeviceID"=w360, "Timestamp"=w365, "MicrogridID"=w364, "Active"=w354, "Inactive"=w363) -> (w323:T16)  [unwired: 3 in]
          n122 = case shown="True" w375 {
            tunnel: w334 -> [w391 w401]
            tunnel: [w391 w394] -> w327
            tunnel: w323 -> [_ w396]
            tunnel: w329 -> [_ w397]
            tunnel: w328 -> [_ w399]
            tunnel: w332 -> [_ w400]
            tunnel: w331 -> [_ w393]
            tunnel: w330 -> [_ w392]
            frame False {
            }
            frame True {
              # "Update at 1 Hz"
              n123 = call "Write Single.vim"("Data Element"=w399, "error in"=w401, "Data DVR"=w400) -> ("dup error out"=w398:errorcluster)  [unwired: 8 in]
              n124 = call "Write Single.vim"("Data Element"=w397, "error in"=w398, "Data DVR"=w393) -> ("dup error out"=w395:errorcluster)  [unwired: 8 in]
              n125 = call "Write Single.vim"("Data Element"=w396, "error in"=w395, "Data DVR"=w392) -> ("dup error out"=w394:errorcluster)  [unwired: 8 in]
            }
          }
          n126 = Divide(x=w353, y=w359) -> (x/y=w358:sgl)
          n127 = Divide(x=w352, y=w359) -> (x/y=w357:sgl)
          n128 = Multiply(x=w371, y=w373) -> (x*y=w340:dbl[])
          n129 = Build Array(w358, w358, w358) -> (w344:sgl[])
          n130 = Build Array(w357, w357, w357) -> (w342:sgl[])
          n131 = Multiply(x=w370, y=w372) -> (x*y=w339:dbl[])
          n132 = To Double Precision Float(number=w344) -> (double precision float=w336:dbl[])
          n133 = To Double Precision Float(number=w342) -> (double precision float=w335:dbl[])
          n134 = Multiply(x=w343, y=w336) -> (x*y=w338:dbl[])
          n135 = Multiply(x=w341, y=w335) -> (x*y=w337:dbl[])
          n136 = call "Elapsed Time3"("Time Target (s)"=0.1) -> ("Time has Elapsed"=w325:bool)  [unwired: 11 in, 7 out]
          n137 = Bundle(cluster=T25 {"DeviceID"="", "Voltage"=[], "Current"=[], "RealPower"=[], "ReactivePower"=[], "LineConfig"=[], "Frequency"=0.0} ("DER_Measurement"), "DeviceID"=w360, "Voltage"=w340, "Current"=w339, "RealPower"=w338, "ReactivePower"=w337, "LineConfig"=w377, "Frequency"=w345) -> (w321:T25)
          n138 = global write "Measurements (Global).vi" "Gen V Meas"(w340) -> ()
          n139 = global write "Measurements (Global).vi" "Gen I Meas"(w339) -> ()
          n140 = global write "Measurements (Global).vi" "Gen P Meas"(w338) -> ()
          n141 = global write "Measurements (Global).vi" "Gen Q Meas"(w337) -> ()
          n142 = local read "Vf Control"() -> (w351:bool)
          n143 = local read "Is VF Device?"() -> (w369:bool)
          n144 = Not(x=w351) -> (.not. x?=w350:bool)
          n145 = Bundle(cluster=T23 {"DeviceID"="", "VFControl"=FALSE, "PControl"=FALSE, "QControl"=FALSE, "PFControl"=FALSE, "PVControl"=FALSE, "Droop"=FALSE, "Unbalanced"=FALSE, "MicrogridVF"=FALSE, "RealDroop(kW)"={"XMin"=0.0, "XMax"=0.0, "YMin"=0.0, "YMax"=0.0}, "ReactiveDroop(kVar)"={"XMin"=0.0, "XMax"=0.0, "YMin"=0.0, "YMax"=0.0}} ("DER_Status"), "DeviceID"=w360, "VFControl"=w351, "PControl"=w350, "QControl"=w350, "PFControl"=w349, "PVControl"=w349, "Droop"=w349, "Unbalanced"=w349, "MicrogridVF"=w369) -> (w319:T23)  [unwired: 2 in]
          n146 = case shown="True" w325 {
            tunnel: w324 -> [_ w388]
            tunnel: w327 -> [w380 w390]
            tunnel: w323 -> [_ w389]
            tunnel: w319 -> [_ w382]
            tunnel: [w380 w381] -> w326
            tunnel: w321 -> [_ w385]
            tunnel: w322 -> [_ w386]
            tunnel: w320 -> [_ w383]
            frame False {
            }
            frame True {
              # "Update at 10 Hz"
              n147 = call "Write Single.vim"("Data Element"=w389, "error in"=w390, "Data DVR"=w388) -> ("dup error out"=w387:errorcluster)  [unwired: 8 in]
              n148 = call "Write Single.vim"("Data Element"=w385, "error in"=w387, "Data DVR"=w386) -> ("dup error out"=w384:errorcluster)  [unwired: 8 in]
              n149 = call "Write Single.vim"("Data Element"=w382, "error in"=w384, "Data DVR"=w383) -> ("dup error out"=w381:errorcluster)  [unwired: 8 in]
            }
          }
        }
        frame "CheckClose" {
          # "Check to see if MicrogridID has been reset to 0, releasing the device from Microgrid control"
          n150 = Select(t=DDS_State."Close", s=FALSE, f=DDS_State."ReadDDS") -> (s? t:f=w424:T2)
        }
        frame "Close" {
          # "Set MicrogridID to 0 in order for Generation Mode Loop to function correctly."
          # "Deactivate the device"
          # "Release resources associated with microgrid ID, deactivate device, and return to CheckID state"
          n151 = flat-sequence {
            frame #0 {
              # "disables output"
              n152 = local write "Enable INV A"(FALSE ("PWM Enabled")) -> ()
            }
          }
          n153 = local write "MicrogridID"(u8 0 ("MicrogridID")) -> ()
        }
        frame "Shutdown" {
          # "Set MicrogridID to 0 in order for Generation Mode Loop to function correctly."
          # "Deactivate the device"
          # "Release resources and stop loop"
          n154 = flat-sequence {
            frame #0 {
              # "disables output"
              n155 = local write "Enable INV A"(FALSE ("PWM Enabled")) -> ()
            }
          }
          n156 = local write "MicrogridID"(u8 0 ("MicrogridID")) -> ()
        }
      }
      "DDS Loop error out" <- w156
      n157 = global read "Stop (Global).vi" "stop"() -> (w140:bool)
      n158 = local read "MicrogridID"() -> (w144:u8)
      n159 = local read "Is VF Device?"() -> (w143:bool)
      n160 = Unbundle By Name(w156) -> ("status"=→"Error in DDS Loop":bool)
      n161 = local read "DDS State"() -> (w142:T2)
      n162 = Wait (ms)(milliseconds to wait=u32 0) -> (millisecond timer value=w152:u32)
      n163 = Or(x=w140, y=w156) -> (x .or. y?=w158:bool)
      n164 = feedback #1() -> (w151:u32)  [unwired: 1 in]
      n165 = feedback-in #1(w152) -> ()
      n166 = Select(t=DDS_State."Shutdown", s=w158, f=w160) -> (s? t:f=w161:T2)
      n167 = Subtract(x=w152, y=w151) -> (x-y=→"DDS loop time":u32)
      n168 = Bundle("DDS State"=w142, "Is VF Device?"=w143, "MicrogridID"=w144) -> (→"DDS Indicators":T3)  [unwired: 1 in]
      "DDS State" <- w139
    }
    n169 = while "Generation Mode Loop" {
      shift-right: [w51] -> _
      shift-left: w30 -> [w54]
      shift-right: [w45] -> w29
      shift-left: errorcluster {"status"=FALSE, "code"=0, "source"=""} ("error out") -> [w49]
      tunnel: w31 -> [w47]
      tunnel: w23 -> [w50]
      stop <- w44 stop-if-true
      # "Handles generation mode switching"
      n170 = case shown="\"VF Device\"" w54 {
        tunnel: [w56 Generation_Mode_Loop_Selector."Active" w73 w96 Generation_Mode_Loop_Selector."VF Device" Generation_Mode_Loop_Selector."Commissioning" Generation_Mode_Loop_Selector."Commissioning"] -> w52
        tunnel: [_ _ _ _ _ _ TRUE] -> w44
        tunnel: w50 -> [_ _ w69 w90 _ _ _]
        tunnel: w49 -> [w55 w62 w68 w91 w132 w134 w137]
        tunnel: [w55 w62 w64 w86 w132 w134 w137] -> w45
        tunnel: w47 -> [_ _ w67 w89 _ _ _]
        frame "Commissioning" {
          # "Start up case that allows DDS State Machine to get a Microgrid ID before going into rest of state machine"
          n171 = Wait (ms)(milliseconds to wait=u32 100) -> ()  [unwired: 1 out]
          n172 = local read "MicrogridID"() -> (w60:u8)
          n173 = Equal To 0?(x=w60) -> (x = 0?=w59:bool)
          n174 = Select(t=Generation_Mode_Loop_Selector."Commissioning", s=w59, f=Generation_Mode_Loop_Selector."Start") -> (s? t:f=w56:T5)
        }
        frame "Start" {
          # "Initialize reader looking at Generation Mode"
        }
        frame "Active" {
          # "Able to switch generation modes, but not available for VF."
          n175 = Unbundle By Name(w69) -> ("DER_setGenerationMode"=w70:refnum<data-value>)
          n176 = Wait (ms)(milliseconds to wait=u32 100) -> ()  [unwired: 1 out]
          n177 = call "Read Single.vim"("Data Type"=T12 {"DeviceID"="", "Mode"=enum."Invalid"} ("DER_setGenerationMode"), "DeviceID"=w67, "error in"=w68, "Data DVR"=w70) -> ("dup error out"=w64:errorcluster, "Valid"=w66:bool, "Data Element"=w65:T12)  [unwired: 5 in]
          n178 = case shown="True" w66 {
            tunnel: w65 -> [_ w82]
            frame False {
            }
            frame True {
              # "DeviceID Match"
              n179 = Unbundle By Name(w82) -> ("Mode"=w81:T13)
              n180 = case shown="\"VF\"" w81 {
                frame "Invalid", Default {
                }
                frame "VF" {
                  # "Added this case for situation where we hot swap VF devices while offgrid.  If this device is no longer the VF device, it gets kicked to \"Active\" case and setGenerationMode flag is probably still \"VF\""
                  n181 = local write "Vf Control"(FALSE ("Vf Control")) -> ()
                }
                frame "PQ" {
                  # "PQ is a valid mode, make sure all settings are correct"
                  n182 = local write "Vf Control"(FALSE ("Vf Control")) -> ()
                }
                frame "Droop" {
                  n183 = local write "Vf Control"(FALSE ("Vf Control")) -> ()
                }
              }
            }
          }
          n184 = local read "Is VF Device?"() -> (w75:bool)
          n185 = Select(t=Generation_Mode_Loop_Selector."VF Device", s=w75, f=Generation_Mode_Loop_Selector."Active") -> (s? t:f=w74:T5)
          n186 = local read "MicrogridID"() -> (w80:u8)
          n187 = Equal To 0?(x=w80) -> (x = 0?=w79:bool)
          n188 = Select(t=Generation_Mode_Loop_Selector."Close References", s=w79, f=w74) -> (s? t:f=w73:T5)
        }
        frame "VF Device" {
          # "Active, plus available for VF mode.."
          n189 = Unbundle By Name(w90) -> ("DER_setGenerationMode"=w92:refnum<data-value>)
          n190 = Wait (ms)(milliseconds to wait=u32 1) -> ()  [unwired: 1 out]
          n191 = call "Read Single.vim"("Data Type"=T12 {"DeviceID"="", "Mode"=enum."Invalid"} ("DER_setGenerationMode"), "DeviceID"=w89, "error in"=w91, "Data DVR"=w92) -> ("dup error out"=w86:errorcluster, "Valid"=w87:bool, "Data Element"=w88:T12)  [unwired: 5 in]
          n192 = case shown="True" w87 {
            tunnel: w88 -> [_ w120]
            tunnel: [Generation_Mode_Loop_Selector."VF Device" w106] -> w94
            frame False {
              n193 = global read "Measurements (Global).vi" "PCC Status"() -> (w104:bool)
              n194 = Not(x=w104) -> (.not. x?=w103:bool)
              n195 = local write "Vf Control"(w103) -> ()
            }
            frame True {
              # "DeviceID Match"
              n196 = Unbundle By Name(w120) -> ("Mode"=w119:T13)
              n197 = feedback #2() -> (w113:T13)  [unwired: 1 in]
              n198 = case shown="\"VF\"" w119 {
                tunnel: w119 -> [_ w124 w126 w129]
                tunnel: [w121 w124 w126 w129] -> w118
                tunnel: w113 -> [w121 _ _ _]
                frame "Invalid", Default {
                }
                frame "PQ" {
                  # "PQ is a valid mode, make sure all settings are correct"
                  n199 = global read "Measurements (Global).vi" "PCC Status"() -> (w123:bool)
                  n200 = Not(x=w123) -> (.not. x?=w122:bool)
                  n201 = local write "Vf Control"(w122) -> ()
                }
                frame "Droop" {
                  n202 = local write "Vf Control"(FALSE ("Vf Control")) -> ()
                }
                frame "VF" {
                  # "Switches device to Voltage-Frequency control"
                  n203 = global read "Measurements (Global).vi" "PCC Status"() -> (w128:bool)
                  n204 = Not(x=w128) -> (.not. x?=w127:bool)
                  n205 = local write "Vf Control"(w127) -> ()
                }
              }
              n206 = feedback-in #2(w118) -> ()
              n207 = Equal?(x=GenerationMode."PQ", y=w118) -> (x = y?=w115:bool)
              n208 = Equal?(x=GenerationMode."Droop", y=w118) -> (x = y?=w114:bool)
              n209 = Equal?(x=GenerationMode."VF", y=w113) -> (x = y?=w110:bool)
              n210 = Or(x=w115, y=w114) -> (x .or. y?=w111:bool)
              n211 = And(x=w111, y=w110) -> (x .and. y?=w109:bool)
              n212 = Select(t=Generation_Mode_Loop_Selector."Hold", s=w109, f=Generation_Mode_Loop_Selector."VF Device") -> (s? t:f=w106:T5)
            }
          }
          n213 = local read "Is VF Device?"() -> (w98:bool)
          n214 = Select(t=w94, s=w98, f=Generation_Mode_Loop_Selector."Active") -> (s? t:f=w97:T5)
          n215 = local read "MicrogridID"() -> (w102:u8)
          n216 = Equal To 0?(x=w102) -> (x = 0?=w101:bool)
          n217 = Select(t=Generation_Mode_Loop_Selector."Close References", s=w101, f=w97) -> (s? t:f=w96:T5)
        }
        frame "Hold" {
          # "Set P and Q setpoints to current values when transitioning from VF to PQ"
          n218 = local read "Q_meas"() -> (w130:sgl)
          n219 = local read "P_meas"() -> (w131:sgl)
          n220 = local write "P_ref"(w131) -> ()
          n221 = local write "Q_ref"(w130) -> ()
        }
        frame "Close References" {
          # "close connection/reference to DDS Reader for DER_setGenerationMode"
        }
        frame "Shutdown" {
          # "Release resources and close loop"
        }
      }
      "error out GenMode Loop" <- w45
      n222 = Unbundle By Name(w45) -> ("status"=→"Error in Generation Mode Loop":bool)
      n223 = Wait (ms)(milliseconds to wait=u32 0) -> (millisecond timer value=w42:u32)
      n224 = global read "Stop (Global).vi" "stop"() -> (w39:bool)
      n225 = feedback #3() -> (w41:u32)  [unwired: 1 in]
      n226 = feedback-in #3(w42) -> ()
      n227 = Or(x=w45, y=w39) -> (x .or. y?=w48:bool)
      n228 = Subtract(x=w42, y=w41) -> (x-y=→"DDS state m/c loop time":u32)
      n229 = Select(t=Generation_Mode_Loop_Selector."Shutdown", s=w48, f=w52) -> (s? t:f=w51:T5)
    }
    "DeviceID" <- w34
  }
  "Q_ref" <- w6
  "P_ref" <- w7
